vi "Test Waveform Diogo backup.vi"() -> ()   [LabVIEW 2016]
uses:
  <vilib>/measure/matone.llb/Extract Single Tone Information 1 Chan.vi
  <vilib>/measure/mamon.llb/Create Continuous Mask.vi
  <vilib>/measure/mamon.llb/Limit Testing Time.vi
  <vilib>/xnet/xnet.llb/XNET Read (Signal Waveform) .vi
  <vilib>/Waveform/WDTOps.llb/WDT Append Waveforms DBL.vi
  <vilib>/Waveform/WDTOps.llb/WDT Number of Waveform Samples DBL.vi
  <vilib>/measure/matone.llb/Extract Single Tone Information N Chan.vi
  <vilib>/measure/NI_MAPro.lvlib
  <vilib>/measure/mamon.llb/Create Continuous Mask using Formula.vi
  <vilib>/measure/NI_MABase.lvlib
  <vilib>/measure/mascope.llb/Pulse Measurements N chan.vi
  <vilib>/measure/mascope.llb/Pulse Measurements 1 chan.vi
panel:
  out "detected frequencies":dbl[](array[numeric]) format="%.2p"
  out "Waveform Graph 3":dynamicdata(graph)
  in  "signal type":T1(ring)
  out "detected amplitude":dbl format="%.2p"
  in  "amplitude":dbl=1.0 format="%0.2p"
  out "test passed?":bool
  out "error out 3":errorcluster
  out "error out 2":errorcluster caption="error out"
  out "error out":errorcluster
  out "Limit 3":cluster{"x0":dbl, "dx":dbl, "Y":dbl[]} caption="Limit" {"Y" format="%.2p"; "dx" format="%.2p"; "x0" format="%.2p"}
  out "detected phase (deg)":dbl format="%.2p"
  out "Waveform Graph 2":waveform(dbl)(graph)
  out "pulse duration 2":dbl format="%.2g"
  out "duty cycle 2":dbl format="%.2g"
  out "measurement info 2":T2 {"ref levels"."ref units" items=["absolute", "relative"]; "ref levels"."high ref level" format="%.2p"; "ref levels"."low ref level" format="%.2p"; "ref levels"."mid ref level" format="%.2p"; "pulse center" format="%.2p"}
  out "period 2":dbl
  out "period":dbl
  out "Limit 2":cluster{"x0":dbl, "dx":dbl, "Y":dbl[]} {"Y" format="%.2p"; "dx" format="%.2p"; "x0" format="%.2p"}
  out "Limit":cluster{"x0":dbl, "dx":dbl, "Y":dbl[]} {"Y" format="%.2p"; "dx" format="%.2p"; "x0" format="%.2p"}
  out "Phase":dbl
  out "measurement info":T2 {"ref levels"."ref units" items=["absolute", "relative"]; "ref levels"."high ref level" format="%.2p"; "ref levels"."low ref level" format="%.2p"; "ref levels"."mid ref level" format="%.2p"; "pulse center" format="%.2p"}
  out "remaining elements":dbl[](array[numeric])
  out "duty cycle":dbl format="%.2g"
  out "pulse duration":dbl format="%.2g"
  out "# elements in queue":i32
  out "Waveform Graph":waveform(dbl)[](graph)
  in  "stop":bool
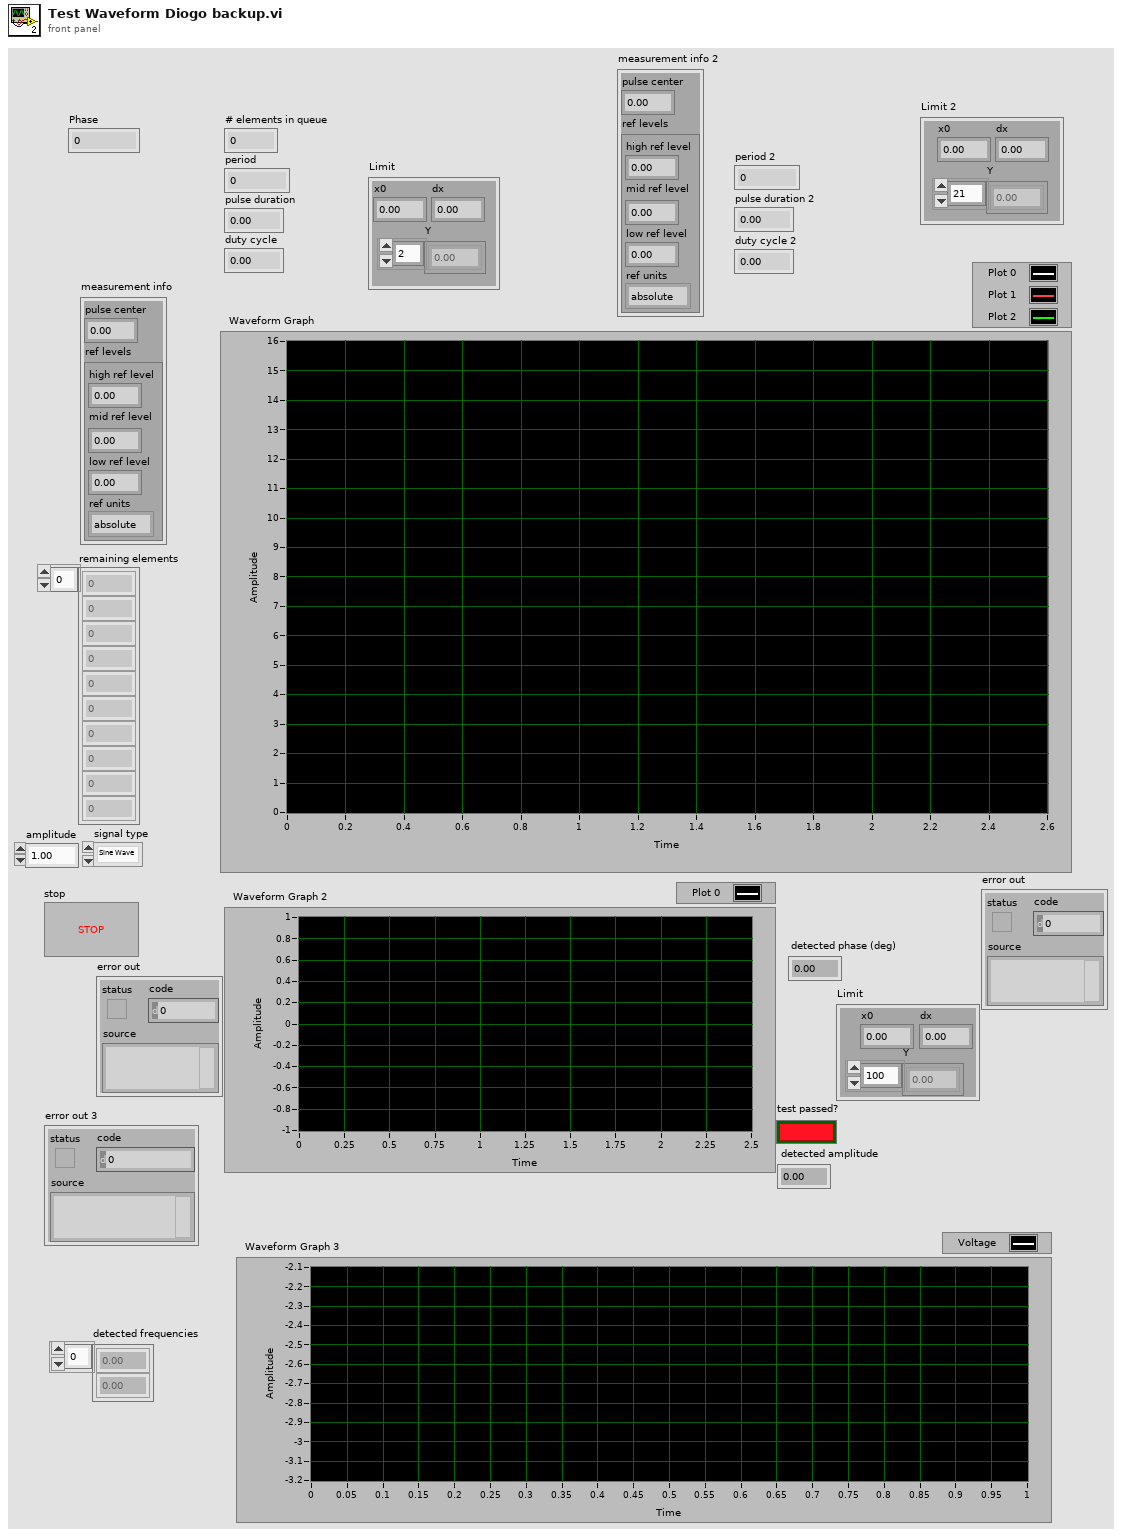
[diagram p1: front panel]
types:
  T1 = enum16{"Sine Wave", "Triangle Wave", "Square Wave", "Sawtooth Wave"}
  T2 = cluster{"pulse center":dbl, "ref levels":cluster{"high ref level":dbl, "mid ref level":dbl, "low ref level":dbl, "ref units":u16}}
  T3 = enum16{"open", "open or create", "create or replace", "create", "open (read-only)"}
  T4 = cluster{"pulse center":dbl, "ref levels":cluster{"high ref level":dbl, "mid ref level":dbl, "low ref level":dbl, "ref units":u16}}[]
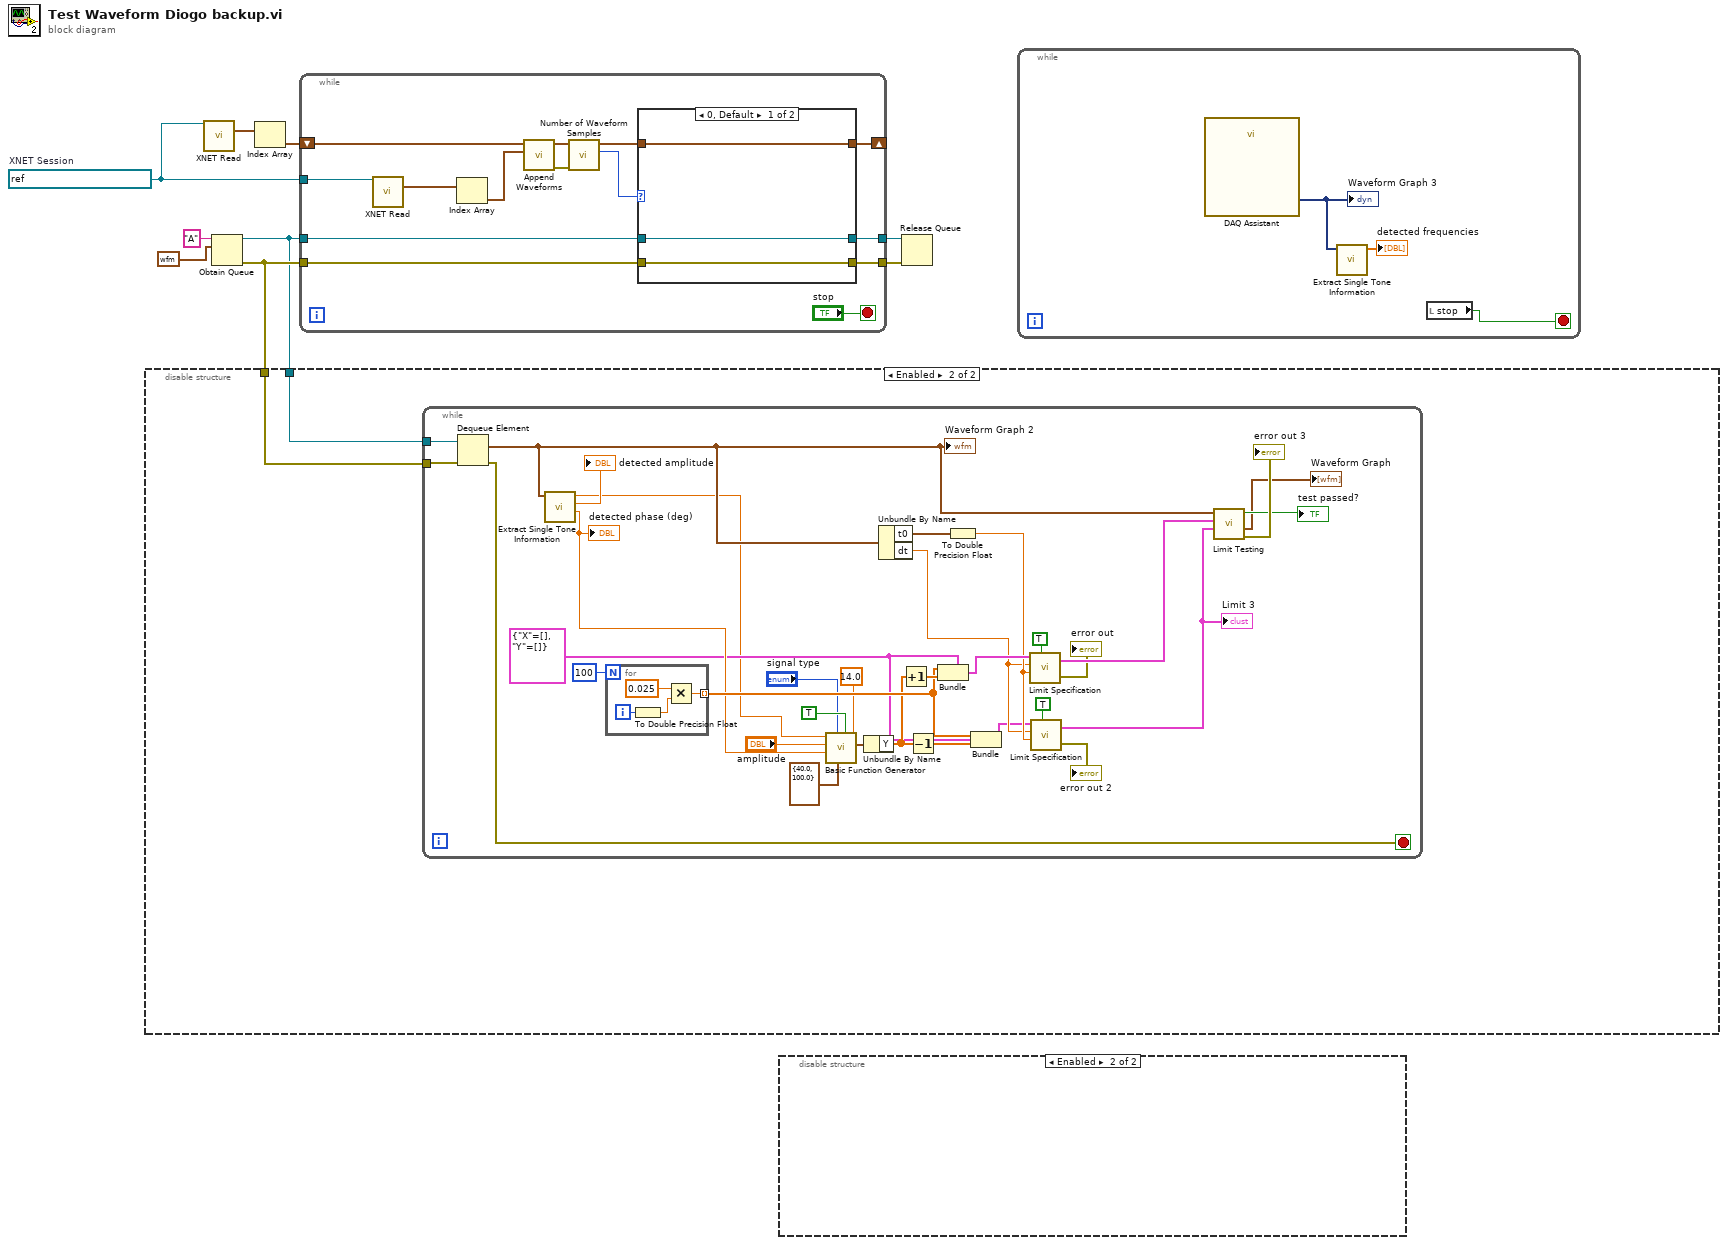
[diagram p0: block diagram]
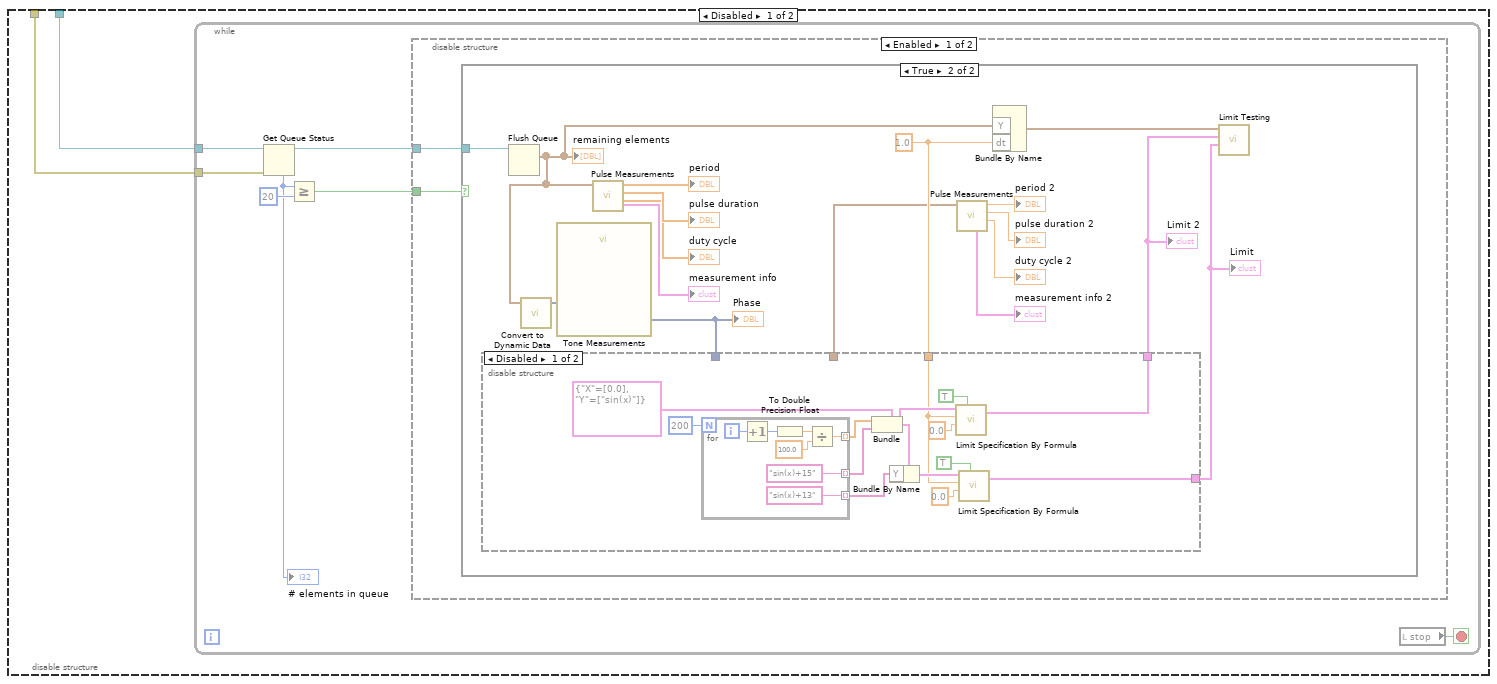
[diagram p2: hidden frame]
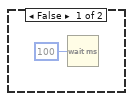
[diagram p3: hidden frame]
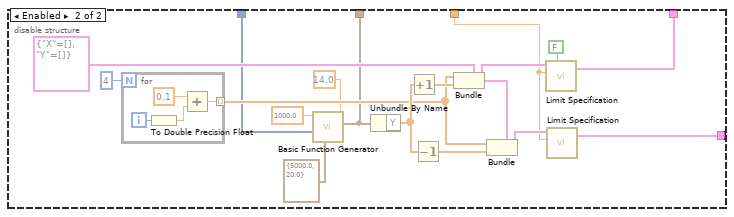
[diagram p4: hidden frame]
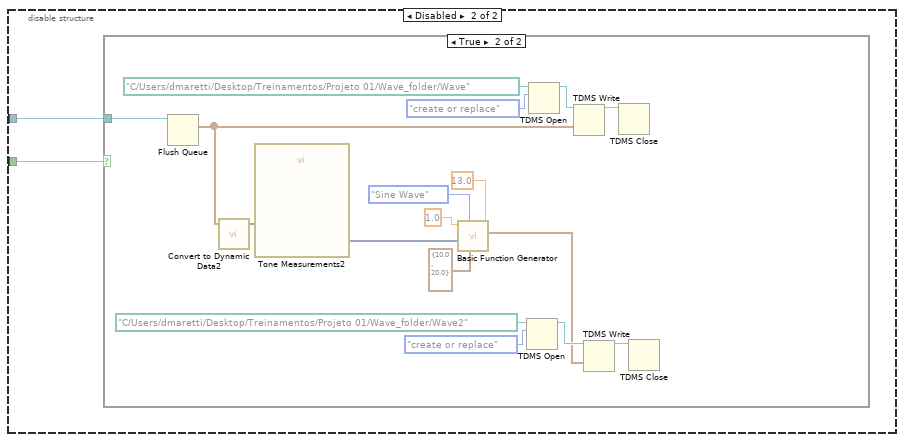
[diagram p5: hidden frame]
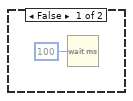
[diagram p6: hidden frame]
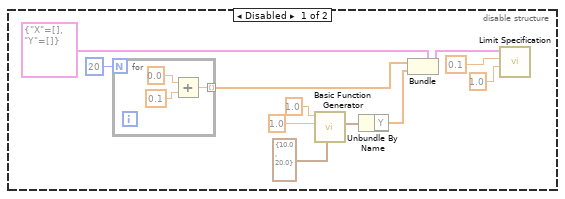
[diagram p7: hidden frame]
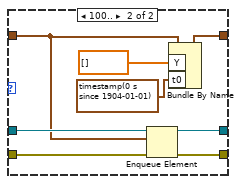
[diagram p8: hidden frame]
diagram:
  w3 = refnum<k21> "New NI-XNET Session"  # XNET Session
  n1 = call-poly <vilib>:"XNET Read.vi"("session in"=w3) -> ("data"=w4:waveform(dbl)[])  [unwired: 12 in, 2 out]
  n2 = Obtain Queue(name (unnamed)="A", element data type=waveform(dbl) {"t0"=timestamp(0 s since 1904-01-01), "dt"=1.0, "Y"=[]}) -> (queue out=w5:refnum<queue>, error out=w6:errorcluster)  [unwired: 3 in, 1 out]
  n3 = disable-structure shown="Enabled" {
    disable-tunnel: w6 -> [w11 w101]
    disable-tunnel: w5 -> [w10 w102]
    frame Disabled {
      n4 = while {
        tunnel: w10 -> [w18]
        tunnel: w11 -> [w17]
        stop <- w14 stop-if-true
        n5 = Get Queue Status(queue=w18, error in (no error)=w17) -> (queue out=w13:refnum<queue>, # elements in queue=w12:i32)  [unwired: 1 in, 6 out]
        "# elements in queue" <- w12
        n6 = Greater Or Equal?(x=w12, y=20) -> (x >= y?=w15:bool)
        n7 = disable-structure shown="Enabled" {
          disable-tunnel: w15 -> [w20 w82]
          disable-tunnel: w13 -> [w19 w81]
          frame Enabled {
            n8 = case shown="True" w20 {
              tunnel: w19 -> [_ w38]
              frame False {
                n9 = Wait (ms)(milliseconds to wait=u32 100) -> ()  [unwired: 1 out]
              }
              frame True {
                w30 = 1.0 ("dt")
                n10 = Flush Queue(queue=w38) -> (remaining elements=w29:waveform(dbl)[])  [unwired: 1 in, 2 out]
                "remaining elements" <- w29
                n11 = call "Convert to Dynamic Data"("Array"=w29) -> ("Dynamic Data Type"=w34:dynamicdata)  [unwired: 3 in]
                n12 = call "Tone Measurements"("Signals"=w34) -> ("Phase"=w27:dynamicdata)  [unwired: 9 in, 1 out]
                "Phase" <- w27
                n13 = disable-structure shown="Disabled" {
                  disable-tunnel: [w44 w68] -> w33
                  disable-tunnel: [w43 w69] -> w32
                  disable-tunnel: w30 -> [w40 w67]
                  disable-tunnel: w27 -> [_ w61]
                  disable-tunnel: [_ w60] -> w22
                  frame Disabled {
                    n14 = for {
                      N: 200 -> [_]
                      tunnel: [w59] -> w39 mode=indexing
                      tunnel: ["sin(x)+15" ("String")] -> w49 mode=indexing
                      tunnel: ["sin(x)+13" ("String")] -> w45 mode=indexing
                      i -> [w56]
                      n15 = Increment(x=w56) -> (x+1=w58:i32)
                      n16 = To Double Precision Float(number=w58) -> (double precision float=w55:dbl)
                      n17 = Divide(x=w55, y=100.0) -> (x/y=w59:dbl)
                    }
                    n18 = Bundle(cluster=cluster{"X":dbl[], "Y":string[]} {"X"=[0.0], "Y"=["sin(x)"]} ("Specification Cluster"), "X"=w39, "Y"=w49) -> (w47:cluster{"X":dbl[], "Y":string[]})
                    n19 = Bundle By Name(cluster=w47, "Y"=w45) -> (w46:cluster{"X":dbl[], "Y":string[]})
                    n20 = call-poly <vilib>:"Limit Specification By Formula.vi"("Specification Cluster"=w47, "dx"=w40, "x0"=0.0, "Reset"=TRUE) -> ("Limit"=w43:cluster{"x0":dbl, "dx":dbl, "Y":dbl[]})  [unwired: 1 in, 1 out]
                    n21 = call-poly <vilib>:"Limit Specification By Formula.vi"("Specification Cluster"=w46, "dx"=w40, "x0"=0.0, "Reset"=TRUE) -> ("Limit"=w44:cluster{"x0":dbl, "dx":dbl, "Y":dbl[]})  [unwired: 1 in, 1 out]
                  }
                  frame Enabled {
                    n22 = for {
                      N: 4 -> [_]
                      tunnel: [w80] -> w65 mode=indexing
                      i -> [w78]
                      n23 = To Double Precision Float(number=w78) -> (double precision float=w77:dbl)
                      n24 = Add(x=0.1 ("y"), y=w77) -> (x+y=w80:dbl)
                    }
                    n25 = call <vilib>:"Basic Function Generator.vi"("offset"=14.0, "sampling info"=cluster{"Fs":dbl, "#s":dbl} {"Fs"=5000.0, "#s"=20.0}, "phase"=w61, "frequency"=1000.0) -> ("signal out"=w60:waveform(dbl))  [unwired: 5 in, 2 out]
                    n26 = Unbundle By Name(w60) -> ("Y"=w72:dbl[])
                    n27 = Increment(x=w72) -> (x+1=w75:dbl[])
                    n28 = Decrement(x=w72) -> (x-1=w71:dbl[])
                    n29 = Bundle(cluster=cluster{"X":dbl[], "Y":dbl[]} {"X"=[], "Y"=[]} ("Specification Cluster"), "X"=w65, "Y"=w75) -> (w73:cluster{"X":dbl[], "Y":dbl[]})
                    n30 = Bundle(cluster=w73, "X"=w65, "Y"=w71) -> (w74:cluster{"X":dbl[], "Y":dbl[]})
                    n31 = call-poly <vilib>:"Limit Specification.vi"("Specification Cluster"=w73, "dx"=w67, "Reset"=FALSE) -> ("Limit"=w69:cluster{"x0":dbl, "dx":dbl, "Y":dbl[]})  [unwired: 2 in, 1 out]
                    n32 = call-poly <vilib>:"Limit Specification.vi"("Specification Cluster"=w74, "dx"=w67) -> ("Limit"=w68:cluster{"x0":dbl, "dx":dbl, "Y":dbl[]})  [unwired: 3 in, 1 out]
                  }
                }
                "Limit" <- w33
                "Limit 2" <- w32
                n33 = call-poly <vilib>:"Pulse Measurements.vi"("signal(s) in"=w29) -> ("duty cycle"=→"duty cycle":dbl[], "pulse duration"=→"pulse duration":dbl[], "period"=→"period":dbl[], "measurement info"=→"measurement info":T4)  [unwired: 6 in, 1 out]
                n34 = call-poly <vilib>:"Pulse Measurements.vi"("signal in"=w22) -> ("duty cycle"=→"duty cycle 2":dbl, "pulse duration"=→"pulse duration 2":dbl, "period"=→"period 2":dbl, "measurement info"=→"measurement info 2":T2)  [unwired: 6 in, 1 out]
                n35 = Bundle By Name("Y"=w29, "dt"=w30) -> (w31:waveform(dbl))  [unwired: 1 in]
                n36 = call-poly <vilib>:"Limit Testing.vi"("lower limit"=w33, "upper limit"=w32, "signal in"=w31) -> ()  [unwired: 3 in, 6 out]
              }
            }
          }
          frame Disabled {
            n37 = case shown="True" w82 {
              tunnel: w81 -> [_ w100]
              frame False {
                n38 = Wait (ms)(milliseconds to wait=u32 100) -> ()  [unwired: 1 out]
              }
              frame True {
                n39 = Flush Queue(queue=w100) -> (remaining elements=w84:waveform(dbl)[])  [unwired: 1 in, 2 out]
                n40 = call "Convert to Dynamic Data2"("Array"=w84) -> ("Dynamic Data Type"=w95:dynamicdata)  [unwired: 3 in]
                n41 = call "Tone Measurements2"("Signals"=w95) -> ("Phase"=w94:dynamicdata)  [unwired: 9 in, 1 out]
                n42 = call <vilib>:"Basic Function Generator.vi"("offset"=13.0, "sampling info"=cluster{"Fs":dbl, "#s":dbl} {"Fs"=10.0, "#s"=20.0}, "signal type"=T1."Sine Wave", "phase"=w94, "frequency"=1.0) -> ("signal out"=w85:waveform(dbl))  [unwired: 4 in, 2 out]
                n43 = TDMS Open(10:T3."create or replace" ("operation (0:open)"), 11:path "C:/Users/dmaretti/Desktop/Treinamentos/Projeto 01/Wave_folder/Wave2" ("file path")) -> (3:w86:refnum<k34>)  [unwired: 5 in, 1 out]
                n44 = TDMS Open(10:T3."create or replace" ("operation (0:open)"), 11:path "C:/Users/dmaretti/Desktop/Treinamentos/Projeto 01/Wave_folder/Wave" ("file path")) -> (3:w99:refnum<k34>)  [unwired: 5 in, 1 out]
                n45 = TDMS Write(0:w99, 9:w84) -> (4:w97:refnum<k34>)  [unwired: 4 in, 3 out]
                n46 = TDMS Write(0:w86, 9:w85) -> (4:w88:refnum<k34>)  [unwired: 4 in, 3 out]
                n47 = TDMS Close(11:w97) -> ()  [unwired: 1 in, 2 out]
                n48 = TDMS Close(11:w88) -> ()  [unwired: 1 in, 2 out]
              }
            }
          }
        }
        n49 = local read "stop"() -> (w14:bool)
      }
    }
    frame Enabled {
      n50 = while {
        tunnel: w102 -> [w135]
        tunnel: w101 -> [w134]
        stop <- w133 stop-if-true
        w107 = cluster{"X":dbl[], "Y":dbl[]} {"X"=[], "Y"=[]} ("Specification Cluster")
        n51 = Dequeue Element(queue=w135, error in (no error)=w134) -> (element=w109:waveform(dbl), error out=w133:errorcluster)  [unwired: 1 in, 2 out]
        "Waveform Graph 2" <- w109
        n52 = call-poly <vilib>:"Extract Single Tone Information.vi"("time signal in"=w109) -> ("detected phase (deg)"=w124:dbl, "detected amplitude"=→"detected amplitude":dbl, "detected frequency"=w103:dbl)  [unwired: 5 in, 3 out]
        "detected phase (deg)" <- w124
        n53 = for {
          N: 100 -> [_]
          tunnel: [w139] -> w127 mode=indexing
          i -> [w137]
          n54 = To Double Precision Float(number=w137) -> (double precision float=w136:dbl)
          n55 = Multiply(x=0.025 ("y"), y=w136) -> (x*y=w139:dbl)
        }
        n56 = call <vilib>:"Basic Function Generator.vi"("offset"=14.0, "reset signal"=TRUE, "sampling info"=cluster{"Fs":dbl, "#s":dbl} {"Fs"=40.0, "#s"=100.0}, "signal type"="signal type", "phase"=w124, "amplitude"="amplitude", "frequency"=w103) -> ("signal out"=w108:waveform(dbl))  [unwired: 2 in, 2 out]
        n57 = Unbundle By Name(w108) -> ("Y"=w111:dbl[])
        n58 = Unbundle By Name(w109) -> ("t0"=w119:timestamp, "dt"=w117:dbl)
        n59 = Increment(x=w111) -> (x+1=w132:dbl[])
        n60 = Decrement(x=w111) -> (x-1=w130:dbl[])
        n61 = Bundle(cluster=w107, "X"=w127, "Y"=w132) -> (w131:cluster{"X":dbl[], "Y":dbl[]})
        n62 = To Double Precision Float(number=w119) -> (double precision float=w118:dbl)
        n63 = Bundle(cluster=w107, "X"=w127, "Y"=w130) -> (w110:cluster{"X":dbl[], "Y":dbl[]})
        n64 = call-poly <vilib>:"Limit Specification.vi"("Specification Cluster"=w131, "dx"=w117, "x0"=w118, "Reset"=TRUE) -> ("Limit"=w123:cluster{"x0":dbl, "dx":dbl, "Y":dbl[]}, "error out"=→"error out":errorcluster)  [unwired: 1 in]
        n65 = call-poly <vilib>:"Limit Specification.vi"("Specification Cluster"=w110, "dx"=w117, "x0"=w118, "Reset"=TRUE) -> ("Limit"=w112:cluster{"x0":dbl, "dx":dbl, "Y":dbl[]}, "error out"=→"error out 2":errorcluster)  [unwired: 1 in]
        "Limit 3" <- w112
        n66 = call-poly <vilib>:"Limit Testing.vi"("lower limit"=w112, "upper limit"=w123, "signal in"=w109) -> ("error out"=→"error out 3":errorcluster, "output values"=→"Waveform Graph":waveform(dbl)[], "test passed?"=→"test passed?":bool)  [unwired: 3 in, 3 out]
      }
    }
  }
  n67 = Index Array(array=w4) -> (element=w2:waveform(dbl))  [unwired: 1 in]
  n68 = while {
    tunnel: w3 -> [w153]
    tunnel: w5 -> [w151]
    tunnel: [w150] -> w9
    tunnel: [w149] -> w1
    tunnel: w6 -> [w148]
    shift-right: [w141] -> _
    shift-left: w2 -> [w140]
    stop <- "stop" stop-if-true
    n69 = call-poly <vilib>:"XNET Read.vi"("session in"=w153) -> ("data"=w147:waveform(dbl)[])  [unwired: 12 in, 2 out]
    n70 = Index Array(array=w147) -> (element=w146:waveform(dbl))  [unwired: 1 in]
    n71 = call-poly <vilib>:"Append Waveforms.vi"("waveform B"=w146, "waveform A"=w140) -> ("error out"=w145:errorcluster, "waveform out"=w144:waveform(dbl))  [unwired: 8 in]
    n72 = call-poly <vilib>:"Number of Waveform Samples.vi"("error in (no error)"=w145, "waveform in"=w144) -> ("number of samples"=w143:i32, "waveform out"=w142:waveform(dbl))  [unwired: 7 in, 1 out]
    n73 = case shown="0, Default" w143 {
      tunnel: w151 -> [w155 w164]
      tunnel: [w155 w163] -> w150
      tunnel: [w154 w162] -> w149
      tunnel: w148 -> [w154 w161]
      tunnel: w142 -> [w156 w160]
      tunnel: [w156 w159] -> w141
      frame 0, Default {
      }
      frame 100.. {
        n74 = Enqueue Element(queue=w164, element=w160, error in (no error)=w161) -> (queue out=w163:refnum<queue>, error out=w162:errorcluster)  [unwired: 1 in, 1 out]
        n75 = Bundle By Name(cluster=w160, "Y"=dbl[] [], "t0"=timestamp(0 s since 1904-01-01)) -> (w159:waveform(dbl))
      }
    }
  }
  n76 = disable-structure shown="Enabled" {
    frame Disabled {
      n77 = for {
        N: 20 -> [_]
        tunnel: [w176] -> w174 mode=indexing
        n78 = Add(x=0.0 ("Numeric"), y=0.1) -> (x+y=w176:dbl)
      }
      n79 = call <vilib>:"Basic Function Generator.vi"("sampling info"=cluster{"Fs":dbl, "#s":dbl} {"Fs"=10.0, "#s"=20.0}, "amplitude"=1.0, "frequency"=1.0) -> ("signal out"=w170:waveform(dbl))  [unwired: 6 in, 2 out]
      n80 = Unbundle By Name(w170) -> ("Y"=w173:dbl[])
      n81 = Bundle(cluster=cluster{"X":dbl[], "Y":dbl[]} {"X"=[], "Y"=[]} ("Specification Cluster"), "X"=w174, "Y"=w173) -> (w172:cluster{"X":dbl[], "Y":dbl[]})
      n82 = call-poly <vilib>:"Limit Specification.vi"("Specification Cluster"=w172, "dx"=0.1, "x0"=1.0) -> ()  [unwired: 2 in, 2 out]
    }
    frame Enabled {
    }
  }
  n83 = Release Queue(queue=w9, error in (no error)=w1) -> ()  [unwired: 1 in, 3 out]
  n84 = while {
    stop <- w181 stop-if-true
    n85 = call "DAQ Assistant"() -> ("data"=w180:dynamicdata)  [unwired: 16 in, 3 out]
    "Waveform Graph 3" <- w180
    n86 = call-poly <vilib>:"Extract Single Tone Information.vi"("time signals in"=w180) -> ("detected frequencies"=→"detected frequencies":dbl[])  [unwired: 5 in, 5 out]
    n87 = local read "stop"() -> (w181:bool)
  }
